vi "nivsfpga_Reference Global.vi"() -> ()   [LabVIEW 2010]
panel:
  out "DMA_READ FIFO":refnum<vi>
  out "DMA_WRITE FIFO":refnum<vi>
  in  "Standard Template Project Item":refnum<vi>
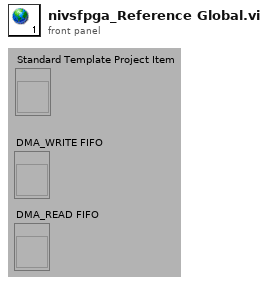
[diagram p1: front panel]
diagram:
